vi "filter.test.vi"(9 "reset":bool, 10 "debug":bool) -> ()   [LabVIEW 2020]
uses:
  <vilib>/Platform/TimedLoop/XDataNode/XDataNode.xnode
  <vilib>/Platform/TimedLoop/XDataNode/nitl_modes.ctl
  <vilib>/Platform/TimedLoop/XDataNode/XDNodeRunTimeDep.lvlib
  <vilib>/Platform/TimedLoop/XDataNode/wakeup.ctl
  <vilib>/Platform/TimedLoop/XDataNode/timing_clust.ctl
  <vilib>/rvi/LocalResourceManager/LocalResourceManager.xnode
  <vilib>/rvi/DataTransferAndStorage/Container/XNode/niFpgaContainer.xnode
  <vilib>/rvi/FIFO/Fifo_Resource/niFpgaFifoEmulationRefIn.vi
  <vilib>/rvi/interface/RandomDataEmulation/nirviRandomDataFpgaMultiElementTemplate.vi
  <vilib>/rvi/FIFO/Fifo_Resource/nirvififoEmulationRead.vi
  ticker.slot.ctl
  Market.Data.Common/fpga/orderbook.command.ctl
  Market.Data.Common/fpga/fpganow.common.fpga.lvlib
  Market.Data.Common/fpga/orderbook.command.type.ctl
  <vilib>/rvi/DataTransferAndStorage/Container/Common/niFpgaContainerGetUniqueNameForEmu.vi
  <vilib>/rvi/DataTransferAndStorage/Container/Common/niFpgaContainerSetEmuInfo.vi
  <vilib>/rvi/eio/common/nirviEmuReportErrorAndStop.vi
  <vilib>/rvi/FIFO/Fifo_Resource/nirvififoEmulationWrite.vi
  <vilib>/rvi/interface/RandomDataEmulation/nirviRandomDataFpgaReadWriteTemplate.vi
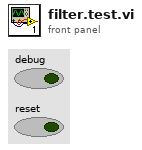
[diagram p1: front panel]
types:
  T1 = typedef "XDNodeRunTimeDep.lvlib/timing_clust.ctl" = cluster{"Expected End [f-1]":u64, "Actual End [f-1]":u64, "Finished Late? [f-1]":bool, "Expected End [i-1]":u64, "Actual End [i-1]":u64, "Finished Late? [i-1]":bool, "Expected Start [i]":u64, "Actual Start [i]":u64, "Expected Start [f]":u64, "Actual Start [f]":u64, "Source Name":string, "Structure Name":string, "Period":i64, "Deadline":i64, "Offset":i64, "Start":i64, "Priority":i32, "Timeout":i32, "Mode":T2, "Wakeup Reason":T3, "Error":errorcluster, "Source Type":string, "Secondary Source Type":string, "Global End Time":u64, "Global Start Time":u64, "Frame Duration":u64, "Iteration Duration":u64, "Assigned CPU":i32, "I/O Scan Engine Mode":u32}
  T2 = typedef "XDNodeRunTimeDep.lvlib/nitl_modes.ctl" = enum32{"No Change", "Process missed periods, maintain original phase", "Discard missed periods, maintain original phase", "Process missed periods, ignore original phase", "Discard missed periods, ignore original phase"}
  T3 = typedef "XDNodeRunTimeDep.lvlib/wakeup.ctl" = enum32{"Normal", "Aborted", "Asynchronous wakeup", "Timing source error", "Timed loop error", "Timeout"}
  T4 = typedef "fpganow.common.fpga.lvlib/orderbook.command.ctl" = cluster{"type":T5, "side":u8, "orderId ":u64, "quantity":u32, "symbol":u64, "price":u64, "executed.qty":u32, "canceled.qty":u32, "remaining.qty":u32, "seconds":u64, "nanoseconds":u64, "Add":bool, "Edit":bool, "Remove":bool, "seq no":u32, "recv.time":u64, "parse.time":u64}
  T5 = typedef "fpganow.common.fpga.lvlib/orderbook.command.type.ctl" = enum8{"Time", "AddOrder", "OrderExecuted", "OrderExecutedAtPrice", "ReduceSize", "ModifyOrder", "DeleteOrder", "Get.Everything", "Get.All.Orders", "Get.Top"}
  T6 = typedef "ticker.slot.ctl" = cluster{"Symbol":u64}
  T7 = cluster{"slot.0":u64, "slot.1":u64, "slot.2":u64, "slot.3":u64}
  T8 = cluster{"type":enum8{"Time", "AddOrder", "OrderExecuted", "OrderExecutedAtPrice", "ReduceSize", "ModifyOrder", "DeleteOrder", "Get.Everything", "Get.All.Orders", "Get.Top"}, "side":u8, "orderId ":u64, "quantity":u32, "symbol":u64, "price":u64, "executed.qty":u32, "canceled.qty":u32, "remaining.qty":u32, "seconds":u64, "nanoseconds":u64, "Add":bool, "Edit":bool, "Remove":bool, "seq no":u32}
  T9 = enum8{"Time", "AddOrder", "OrderExecuted", "OrderExecutedAtPrice", "ReduceSize", "ModifyOrder", "DeleteOrder", "Get.Everything", "Get.All.Orders", "Get.Top"}
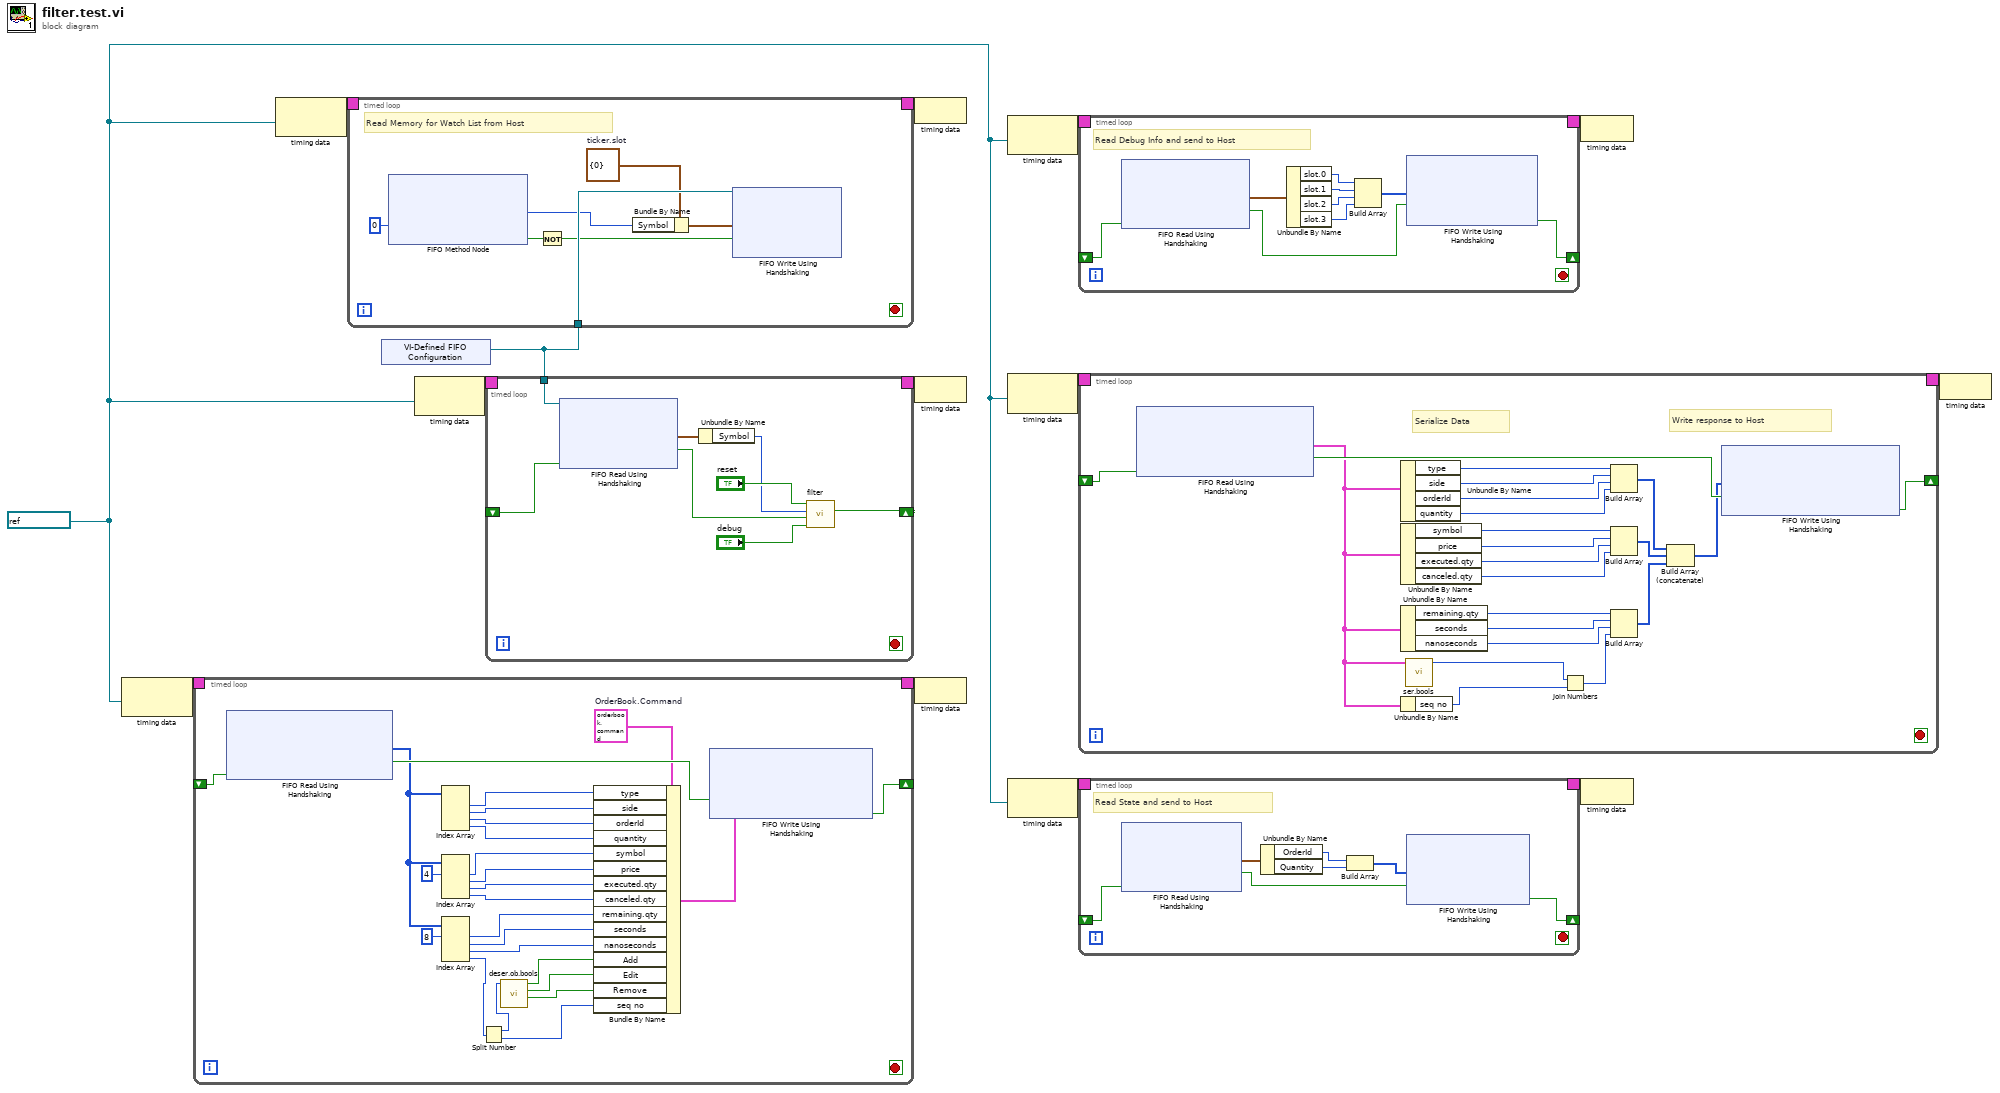
[diagram p0: block diagram]
diagram:
  w1 = refnum<k21> "140MHz" ("Source Name")
  n1 = node-c288(w1) -> (w7:T1)
  n2 = timed-loop {
    timing: w7 -> [_]
    timing-out: [_] -> w6
    shift-right: [w39] -> _
    shift-left: _ -> [w38]
    stop <- _ stop-if-true
    w36 = T4 {"type"=enum."AddOrder", "side"=0, "orderId "=0, "quantity"=0, "symbol"=0, "price"=0, "executed.qty"=0, "canceled.qty"=0, "remaining.qty"=0, "seconds"=0, "nanoseconds"=0, "Add"=FALSE, "Edit"=FALSE, "Remove"=FALSE, "seq no"=0, "recv.time"=0, "parse.time"=0}  # OrderBook.Command
    n3 = xnode ("FIFO Read Using Handshaking")("Ready for Output"=w38) -> ("Element"=w34:u64[], "Output Valid"=w37:bool)  [unwired: 1 in, 1 out]
    n4 = Index Array(array=w34) -> (element #1=w31:u64, element #2=w30:u64, element #3=w29:u64, element #4=w28:u64)  [unwired: 4 in]
    n5 = Index Array(array=w34, index #1=4 ("index")) -> (element #1=w27:u64, element #2=w26:u64, element #3=w25:u64, element #4=w24:u64)  [unwired: 3 in]
    n6 = Index Array(array=w34, index #1=8 ("index")) -> (element #1=w23:u64, element #2=w22:u64, element #3=w21:u64, element #4=w17:u64)  [unwired: 3 in]
    n7 = Split Number(x=w17) -> (hi(x)=w16:u32, lo(x)=w15:u32)
    n8 = call "deser.ob.bools.vi"("Numeric"=w16) -> ("Remove"=w20:bool, "Edit"=w19:bool, "Add"=w18:bool)  [unwired: 8 in]
    n9 = Bundle By Name(cluster=w36, "type"=w31, "side"=w30, "orderId"=w29, "quantity"=w28, "symbol"=w27, "price"=w26, "executed.qty"=w25, "canceled.qty"=w24, "remaining.qty"=w23, "seconds"=w22, "nanoseconds"=w21, "Add"=w18, "Edit"=w19, "Remove"=w20, "seq no"=w15) -> (w35:T4)
    n10 = xnode ("FIFO Write Using Handshaking")("Element"=w35, "Input Valid"=w37) -> ("Ready for Input"=w39:bool)  [unwired: 1 in, 1 out]
  }
  n11 = node-c288(w1) -> (w12:T1)
  n12 = xnode "VI-Defined FIFO Configuration"() -> ("FIFO Out"=w10:refnum<k21>)
  n13 = timed-loop {
    timing: w12 -> [_]
    timing-out: [_] -> w11
    tunnel: w10 -> [w47]
    stop <- _ stop-if-true
    w44 = T6 {"Symbol"=0}  # ticker.slot
    # "Read Memory for Watch List from Host"
    n14 = xnode ("FIFO Method Node")("Timeout"=0) -> ("Element"=w42:u64, "Timed Out?"=w46:bool)  [unwired: 1 in, 1 out]
    n15 = Not(x=w46) -> (.not. x?=w45:bool)
    n16 = Bundle By Name(cluster=w44, "Symbol"=w42) -> (w43:T6)
    n17 = xnode ("FIFO Write Using Handshaking")("Element"=w43, "Input Valid"=w45, "FIFO In"=w47) -> ()  [unwired: 2 out]
  }
  n18 = node-c288(w1) -> (w14:T1)
  n19 = timed-loop {
    timing: w14 -> [_]
    timing-out: [_] -> w13
    tunnel: w10 -> [w58]
    shift-right: [w53] -> _
    shift-left: _ -> [w52]
    stop <- _ stop-if-true
    n20 = xnode ("FIFO Read Using Handshaking")("Ready for Output"=w52, "FIFO In"=w58) -> ("Element"=w57:cluster{"Symbol":u64}, "Output Valid"=w55:bool)  [unwired: 1 out]
    n21 = Unbundle By Name(w57) -> ("Symbol"=w51:u64)
    n22 = call "filter.vi"("debug"="debug", "conf.valid"=w55, "conf"=w51, "reset"="reset") -> ("Ready.for.Configuration.Input"=w53:bool)  [unwired: 6 in, 1 out]
  }
  n23 = node-c288(w11) -> ()
  n24 = node-c288(w13) -> ()
  n25 = node-c288(w6) -> ()
  n26 = node-c288(w1) -> (w9:T1)
  n27 = node-c288(w1) -> (w5:T1)
  n28 = node-c288(w1) -> (w3:T1)
  n29 = timed-loop {
    timing: w9 -> [_]
    timing-out: [_] -> w8
    shift-right: [w69] -> _
    shift-left: _ -> [w68]
    stop <- _ stop-if-true
    # "Read Debug Info and send to Host"
    n30 = xnode ("FIFO Read Using Handshaking")("Ready for Output"=w68) -> ("Element"=w67:T7, "Output Valid"=w61:bool)  [unwired: 1 in, 1 out]
    n31 = Unbundle By Name(w67) -> ("slot.0"=w65:u64, "slot.1"=w66:u64, "slot.2"=w63:u64, "slot.3"=w62:u64)
    n32 = Build Array(w65, w66, w63, w62) -> (w64:u64[])
    n33 = xnode ("FIFO Write Using Handshaking")("Element"=w64, "Input Valid"=w61) -> ("Ready for Input"=w69:bool)  [unwired: 1 in, 1 out]
  }
  n34 = timed-loop {
    timing: w5 -> [_]
    timing-out: [_] -> w4
    shift-right: [w93] -> _
    shift-left: _ -> [w88]
    stop <- _ stop-if-true
    # "Serialize Data"
    # "Write response to Host"
    n35 = xnode ("FIFO Read Using Handshaking")("Ready for Output"=w88) -> ("Element"=w75:T8, "Output Valid"=w87:bool)  [unwired: 1 in, 1 out]
    n36 = Unbundle By Name(w75) -> ("type"=w79:T9, "side"=w78:u8, "orderId"=w77:u64, "quantity"=w76:u32)
    n37 = Unbundle By Name(w75) -> ("symbol"=w92:u64, "price"=w91:u64, "executed.qty"=w90:u32, "canceled.qty"=w89:u32)
    n38 = Unbundle By Name(w75) -> ("remaining.qty"=w83:u32, "seconds"=w81:u64, "nanoseconds"=w82:u64)
    n39 = Unbundle By Name(w75) -> ("seq no"=w74:u32)
    n40 = call "ser.bools.vi"("orderbook.command"=w75) -> ("Numeric"=w73:u32)  [unwired: 10 in]
    n41 = Join Numbers(hi=w73, lo=w74) -> ((hi.lo)=w72:u64)
    n42 = Build Array(w79, w78, w77, w76) -> (w80:u64[])
    n43 = Build Array(w92, w91, w90, w89) -> (w86:u64[])
    n44 = Build Array(w83, w81, w82, w72) -> (w84:u64[])
    n45 = Build Array (concatenate)(w80, w86, w84) -> (w85:u64[])
    n46 = xnode ("FIFO Write Using Handshaking")("Element"=w85, "Input Valid"=w87) -> ("Ready for Input"=w93:bool)  [unwired: 1 in, 1 out]
  }
  n47 = timed-loop {
    timing: w3 -> [_]
    timing-out: [_] -> w2
    shift-right: [w102] -> _
    shift-left: _ -> [w101]
    stop <- _ stop-if-true
    # "Read State and send to Host"
    n48 = xnode ("FIFO Read Using Handshaking")("Ready for Output"=w101) -> ("Element"=w99:cluster{"OrderId":u64, "Quantity":u64}, "Output Valid"=w100:bool)  [unwired: 1 in, 1 out]
    n49 = Unbundle By Name(w99) -> ("OrderId"=w98:u64, "Quantity"=w96:u64)
    n50 = Build Array(w98, w96) -> (w97:u64[])
    n51 = xnode ("FIFO Write Using Handshaking")("Element"=w97, "Input Valid"=w100) -> ("Ready for Input"=w102:bool)  [unwired: 1 in, 1 out]
  }
  n52 = node-c288(w8) -> ()
  n53 = node-c288(w2) -> ()
  n54 = node-c288(w4) -> ()
